vi "_wmg_downlistValue.vi"(1 "Customer":string, 2 "CustomerRef":refnum<vi>) -> ()   [LabVIEW 2011]
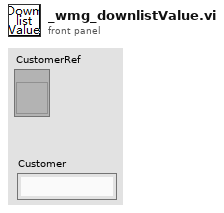
[diagram p1: front panel]
types:
  T1 = typedef "LVStringsAndValuesArrayTypeDef.ctl" = cluster{"String":string, "Value":u16}[]
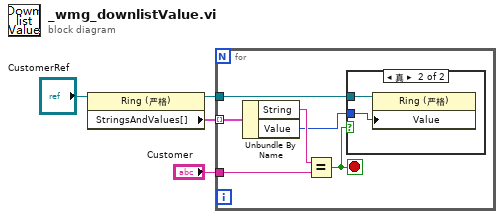
[diagram p0: block diagram]
diagram:
  n1 = property class="Ring (严格)"(reference="CustomerRef") -> (reference out=w2:refnum<vi>, "StringsAndValues[]"=w4:T1)  [unwired: 1 in, 1 out]
  n2 = for {
    tunnel: w4 -> [w10] mode=indexing
    tunnel: "Customer" -> [w8]
    tunnel: w2 -> [w6]
    stop <- w7 stop-if-true
    n3 = Unbundle By Name(w10) -> ("String"=w9:string, "Value"=w5:u16)
    n4 = Equal?(x=w9, y=w8) -> (x = y?=w7:bool)
    n5 = case shown="真" w7 {
      tunnel: w6 -> [_ w12]
      tunnel: w5 -> [_ w11]
      frame False {
      }
      frame True {
        n6 = property class="Ring (严格)"(reference=w12, "Value"=w11) -> ()  [unwired: 1 in, 2 out]
      }
    }
  }
